vi "2D Barcode Add 1 fro Flow Number.vi"(11 "Flow Num":string) -> (3 "Add 1":string)   [LabVIEW 2021]
panel:
  in  "length":i32
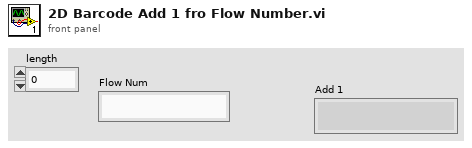
[diagram p1: front panel]
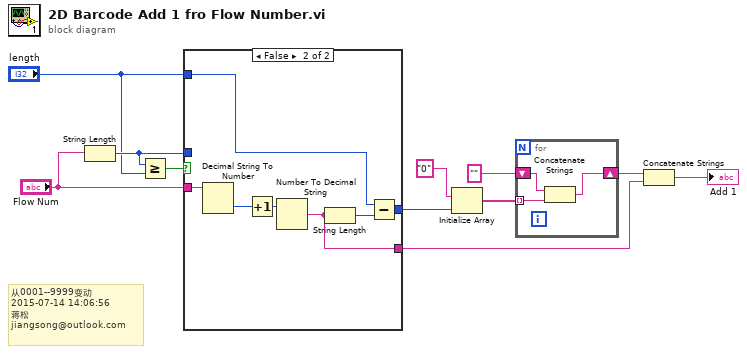
[diagram p0: block diagram]
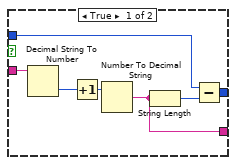
[diagram p2: hidden frame]
diagram:
  # "从0001--9999变动\n2015-07-14 14:06:56\n蒋松\njiangsong@outlook.com"
  n1 = String Length(string="Flow Num") -> (length=w3:i32)
  n2 = Greater Or Equal?(x=w3, y="length") -> (x >= y?=w2:bool)
  n3 = case shown="False" w2 {
    tunnel: [w18 w25] -> w10
    tunnel: [w17 w24] -> w6
    tunnel: "Flow Num" -> [w16 w23]
    tunnel: w3 -> [w12 _]
    tunnel: "length" -> [_ w19]
    frame True {
      n4 = Decimal String To Number(string=w16) -> (number=w15:i32)  [unwired: 2 in, 1 out]
      n5 = Increment(x=w15) -> (x+1=w14:i32)
      n6 = Number To Decimal String(number=w14) -> (decimal integer string=w17:string)  [unwired: 1 in]
      n7 = String Length(string=w17) -> (length=w13:i32)
      n8 = Subtract(x=w12, y=w13) -> (x-y=w18:i32)
    }
    frame False {
      n9 = Decimal String To Number(string=w23) -> (number=w22:i32)  [unwired: 2 in, 1 out]
      n10 = Increment(x=w22) -> (x+1=w21:i32)
      n11 = Number To Decimal String(number=w21) -> (decimal integer string=w24:string)  [unwired: 1 in]
      n12 = String Length(string=w24) -> (length=w20:i32)
      n13 = Subtract(x=w19, y=w20) -> (x-y=w25:i32)
    }
  }
  n14 = Initialize Array("0" ("substring"), w10) -> (w9:string[])
  n15 = for {
    tunnel: w9 -> [w28] mode=indexing
    shift-right: [w26] -> w7
    shift-left: "" ("s? t:f") -> [w27]
    n16 = Concatenate Strings(w27, w28) -> (w26:string)
  }
  n17 = Concatenate Strings(w7, w6) -> (→"Add 1":string)
